vi "xmlStringReadString.vi"(4 "String":string) -> (1 "Value":string)   [LabVIEW 2012]
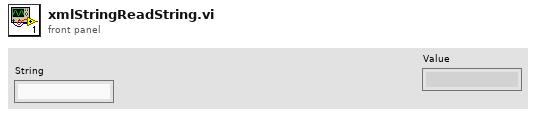
[diagram p1: front panel]
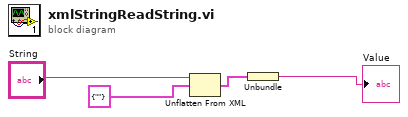
[diagram p0: block diagram]
diagram:
  n1 = Unflatten From XML(xml string="String", type=cluster{string} {""}) -> (value=w3:cluster{string})  [unwired: 1 in, 1 out]
  n2 = Unbundle(w3) -> (→"Value":string)
